vi "DriveModuleControl_TravTunePID.vi"(8 "error in":errorcluster, 9 "Actual State":T1={"Speed"=0.0, "Angle"={"VALUE"=0.0, "COS"=1.0, "SIN"=0.0}} {"Angle"."SIN" format="%13.4f"; "Angle"."COS" format="%13.4f"; "Angle"."VALUE" format="%13.4f"}, 10 "Desired State":T1={"Speed"=0.0, "Angle"={"VALUE"=0.0, "COS"=1.0, "SIN"=0.0}} {"Angle"."SIN" format="%13.4f"; "Angle"."COS" format="%13.4f"; "Angle"."VALUE" format="%13.4f"}, 11 "ModualNamePrefix":i32) -> (0 "error out":errorcluster)   [LabVIEW 2023]
uses:
  <vilib>/Rock Robotics/WPI/ThirdParty/JAS_Junk/TrajLib/TypeDef/SWERVE_DRIVE_MODULE_STATE.ctl
  <vilib>/Rock Robotics/WPI/ThirdParty/JAS_Junk/TrajLib/TypeDef/ROTATION2D.ctl
  <vilib>/Rock Robotics/WPI/ThirdParty/JAS_Junk/TrajLib/Rotation2d_Minus.vi
  <vilib>/Rock Robotics/WPI/ThirdParty/JAS_Junk/TrajLib/Rotation2d_GetRadians.vi
  <vilib>/Rock Robotics/WPI/ThirdParty/JAS_Junk/TrajLib/SwerveModuleState_New.vi
  <vilib>/Rock Robotics/WPI/ThirdParty/JAS_Junk/TrajLib/Rotation2d_RotateBy.vi
  <vilib>/Rock Robotics/WPI/ThirdParty/JAS_Junk/TrajLib/Rotation2d_CreateAngle.vi
  <vilib>/Rock Robotics/WPI/ThirdParty/JAS_Junk/TrajLib/SimpleMotorFF_Calculate.vi
  <vilib>/Rock Robotics/WPI/ThirdParty/JAS_Junk/TrajLib/PIDController_AtSetpoint.vi
  <vilib>/Rock Robotics/WPI/ThirdParty/JAS_Junk/TrajLib/PIDController_SetPIDF.vi
  <vilib>/Rock Robotics/WPI/ThirdParty/JAS_Junk/TrajLib/PIDController_SetDerivativeFilter.vi
  <vilib>/Rock Robotics/WPI/ThirdParty/JAS_Junk/TrajLib/PIDController_SetIntegratorRange.vi
  <vilib>/Rock Robotics/WPI/ThirdParty/JAS_Junk/TrajLib/PIDController_SetTolerancePandV.vi
  <vilib>/Rock Robotics/WPI/ThirdParty/JAS_Junk/TrajLib/PIDController_DisableContinousInput.vi
  <vilib>/Rock Robotics/WPI/ThirdParty/JAS_Junk/TrajLib/PIDController_EnableContinousInput.vi
  <vilib>/Rock Robotics/WPI/ThirdParty/JAS_Junk/TrajLib/PIDController_Reset.vi
  <vilib>/Rock Robotics/WPI/ThirdParty/JAS_Junk/TrajLib/PIDController_New.vi
  <vilib>/Rock Robotics/WPI/ThirdParty/JAS_Junk/TrajLib/PIDController_SetOutputLimits.vi
  <vilib>/Rock Robotics/WPI/ThirdParty/JAS_Junk/TrajLib/Rotation2d_UnaryMinus.vi
  <vilib>/Rock Robotics/WPI/ThirdParty/JAS_Junk/TrajLib/Rotation2d_CreateXY.vi
  <vilib>/Rock Robotics/WPI/ThirdParty/JAS_Junk/TrajLib/PIDController_NewPeriod.vi
  <vilib>/Rock Robotics/WPI/ThirdParty/JAS_Junk/TrajLib/Util_CalcDist.vi
  <vilib>/Rock Robotics/SystemInterfaces/NetworkCommunication/NetComm_UsageReport_report.vi
  DriveGlobal.vi
  <vilib>/Rock Robotics/WPI/ThirdParty/JAS_Junk/TrajLib/Globals/Util_LibraryGlobals.vi
  <vilib>/Rock Robotics/WPI/ThirdParty/JAS_Junk/TrajLib/PIDController_AdvCalculate_FF_Sp_Pv.vi
  <vilib>/Rock Robotics/Network Tables/NT Write Number.vi
  <vilib>/Rock Robotics/WPI/ThirdParty/JAS_Junk/TrajLib/Trajectory_Library.lvlib
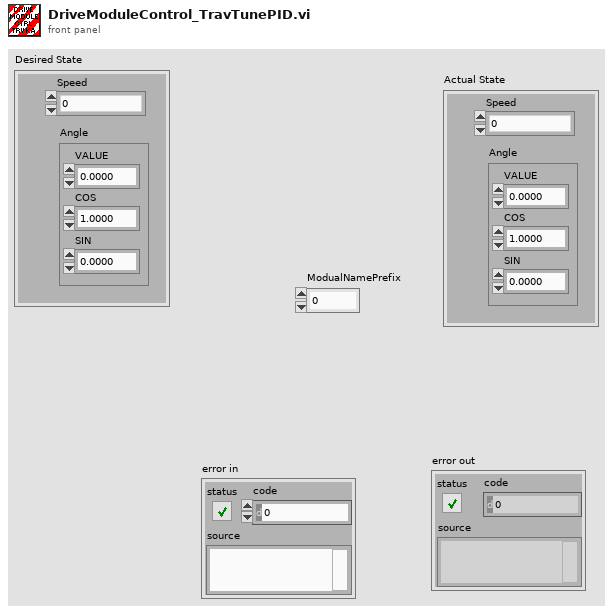
[diagram p1: front panel]
types:
  T1 = typedef "Trajectory_Library.lvlib/SWERVE_DRIVE_MODULE_STATE.ctl" = cluster{"Speed":dbl, "Angle":T2}
  T2 = typedef "Trajectory_Library.lvlib/ROTATION2D.ctl" = cluster{"VALUE":dbl, "COS":dbl, "SIN":dbl}
  T3 = enum16{"Ziegler Nicols - Fast", "Ziegler Nicols - Normal", "Ziegler Nicols - Slow", "CHR regulator - 0% overshoot", "CHR regulator - 20% overshoot", "CHR servo - 0 % overshoot", "CHR servo - 20% overshoot"}
  T4 = typedef "WPI_MotorControlDeviceRef.ctl" = cluster{"DeviceStatus":errorcluster, "Type":T5, "PWM":cluster{"PWM Channel":T6, "DeadBand":T7}, "CAN":cluster{"Device Number":u8, "SetOutput VI Ref":variant, "GetOutput VI Ref":variant, "Enable VI Ref":variant, "Disable VI Ref":variant, "Data":variant}, "Invert":bool, "DIO PWM":cluster{"PWM \"Enable\" Channel":T6, "DIOChannel":T8, "PWM Rate":dbl}}
  T5 = typedef "WPI_MotorControlType.ctl" = enum16{"PWM", "CAN", "DIO PWM"}
  T6 = typedef "FPGA_DIOPWMChannel.ctl" = enum8{"PWM 0", "PWM 1", "PWM 2", "PWM 3", "PWM 4", "PWM 5", "PWM 6", "PWM 7", "PWM 8", "PWM 9", "PWM MXP 0", "PWM MXP 1", "PWM MXP 2", "PWM MXP 3", "PWM MXP 4", "PWM MXP 5", "PWM MXP 6", "PWM MXP 7", "PWM MXP 8", "PWM MXP 9", "Invalid"}
  T7 = typedef "WPI_PWMDeadband.ctl" = cluster{"Name":string, "maxPositivePwm":i32, "minPositivePwm":i32, "centerPwm":i32, "maxNegativePwm":i32, "minNegativePwm":i32, "angularRange":u16}
  T8 = typedef "FPGA_DIOChannel.ctl" = enum8{"DIO 0", "DIO 1", "DIO 2", "DIO 3", "DIO 4", "DIO 5", "DIO 6", "DIO 7", "DIO 8", "DIO 9", "DIO MXP 0", "DIO MXP 1", "DIO MXP 2", "DIO MXP 3", "DIO MXP 4", "DIO MXP 5", "DIO MXP 6", "DIO MXP 7", "DIO MXP 8", "DIO MXP 9", "DIO MXP 10", "DIO MXP 11", "DIO MXP 12", "DIO MXP 13", "DIO MXP 14", "DIO MXP 15", "SPI Port CS1", "SPI Port CS2", "SPI Port CS3", "SPI Port MISO", "SPI Port MOSI", "Invalid"}
  T9 = typedef "Trajectory_Library.lvlib/SIMPLE_MOTOR_FF.ctl" = cluster{"Ks":dbl, "Kv":dbl, "Ka":dbl, "KnInv":dbl}
  T10 = typedef "Trajectory_Library.lvlib/PID_ADV_LIMITS.ctl" = cluster{"MaxInput":dbl, "MinInput":dbl, "Continuous":bool, "MaxOutput":dbl, "MinOutput":dbl}
  T11 = typedef "Trajectory_Library.lvlib/PID_ADV_TUNING.ctl" = cluster{"Kf":dbl, "Kp":dbl, "Ki":dbl, "Kd":dbl, "MaximumIntegral":dbl, "MinimumIntegral":dbl, "Filter Derivative":bool}
  T12 = cluster{"Controller Constant Type":enum16{"Ziegler Nicols - Fast", "Ziegler Nicols - Normal", "Ziegler Nicols - Slow", "CHR regulator - 0% overshoot", "CHR regulator - 20% overshoot", "CHR servo - 0 % overshoot", "CHR servo - 20% overshoot"}, "Type of Controller":enum16{"P", "PI", "PID"}, "CO Offset":dbl, "Kn":dbl, "Tuning Tolerance":dbl, "Plant Tolerance":dbl, "Newest Avg Time ":i32, "Long Ave Time":i32}
  T13 = cluster{"Plant Gain (K)":dbl, "Time Constant (T)":dbl, "Dead Time (L)":dbl, "stimulus operating point":dbl, "response operating point":dbl}
  T14 = cluster{"proportional gain (Kp)":dbl, "integral time (Ki / Sec)":dbl, "derivative time (Kd /Sec)":dbl}
  T15 = cluster{"Const Done":bool, "Plant Done":bool, "PV Std Dev":dbl, "CO Std Dev":dbl}
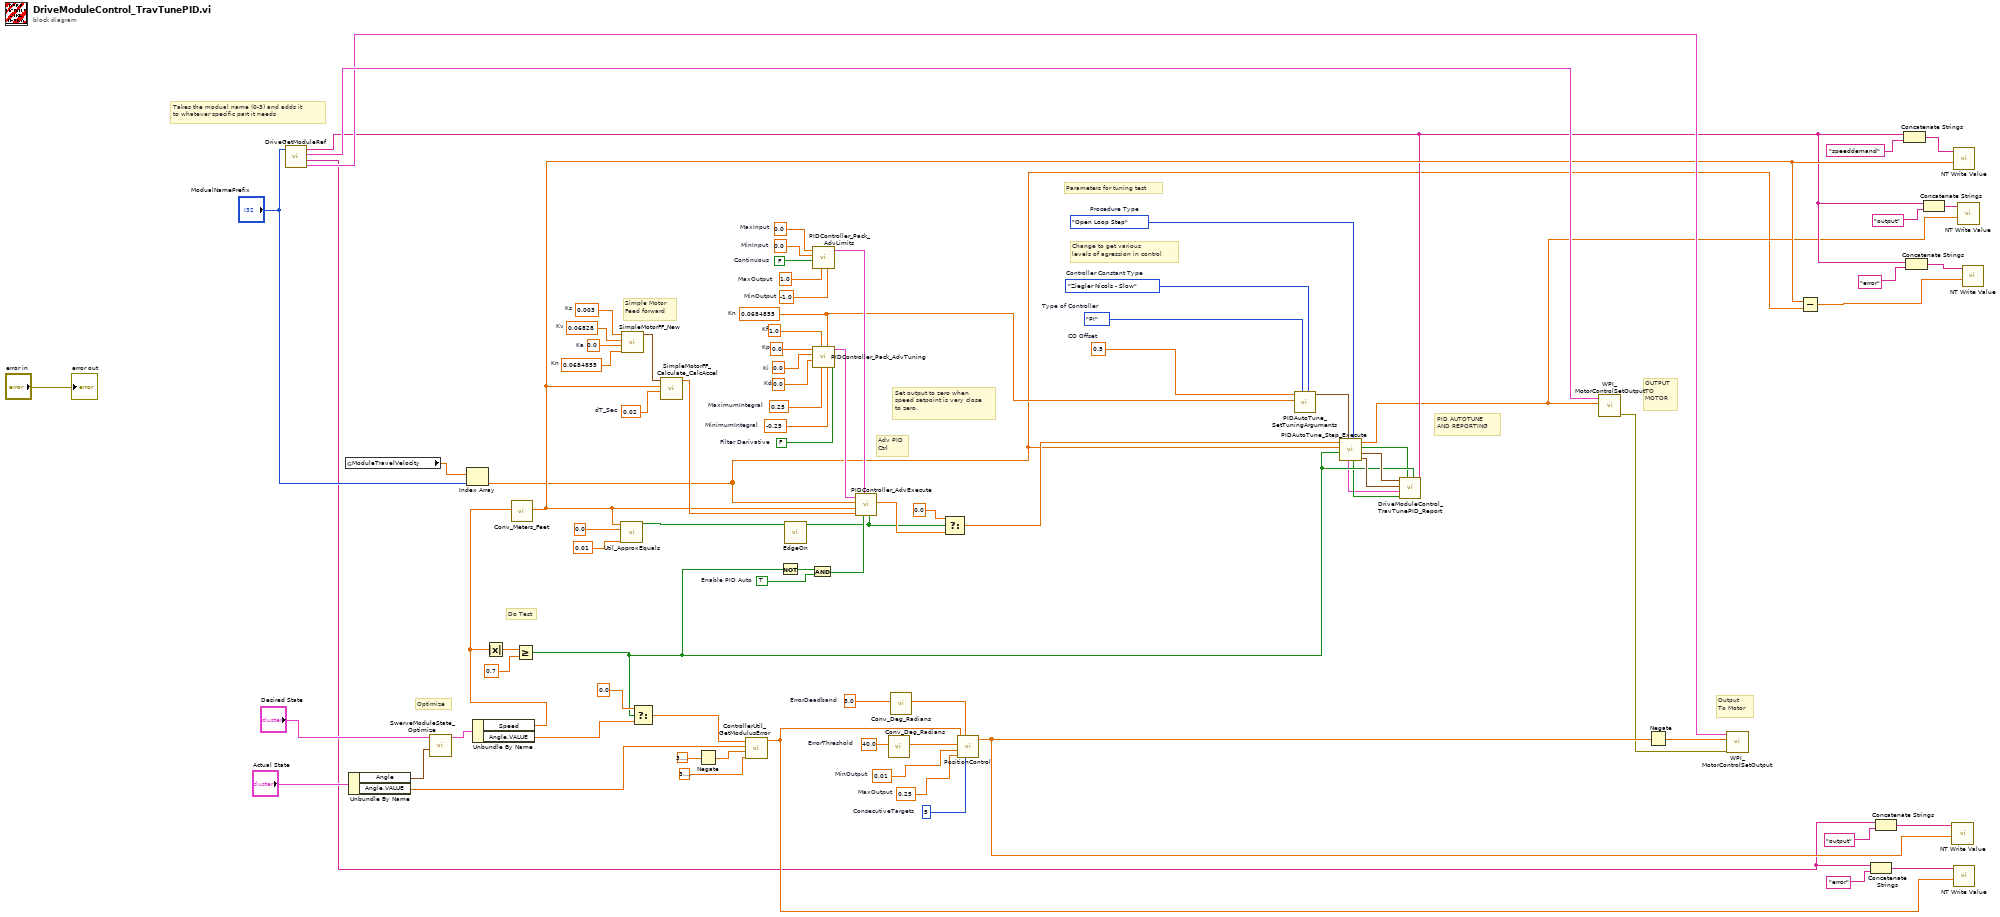
[diagram p0: block diagram]
diagram:
  w12 = enum16{"Open Loop Step", "Closed Loop Step"}."Open Loop Step"  # Procedure Type
  w13 = T3."Ziegler Nicols - Slow"  # Controller Constant Type
  w14 = enum16{"P", "PI", "PID"}."PI"  # Type of Controller
  w15 = 0.5  # CO Offset
  w27 = TRUE  # Enable PID Auto
  w11 = 0.0684855  # Kn
  w53 = 0.0  # Kp
  w52 = 0.0  # Ki
  w51 = 0.0  # Kd
  w50 = 1.0  # Kf
  w49 = 0.25  # MaximumIntegral
  w48 = -0.25  # MinimumIntegral
  w47 = FALSE  # Filter Derivative
  w45 = 0.0  # MinInput
  w44 = FALSE  # Continuous
  w43 = 1.0  # MaxOutput
  w46 = -1.0  # MinOutput
  w42 = 0.0  # MaxInput
  w62 = 0.0684855  # Kn
  w61 = 0.02  # dT_Sec
  w59 = 0.003  # Ks
  w58 = 0.06828  # Kv
  w57 = 0.0  # Ka
  w72 = 5  # ConsecutiveTargets
  w69 = 0.25  # MaxOutput
  w73 = 0.01  # MinOutput
  w66 = 40.0  # ErrorThreshold
  w68 = 3.0  # ErrorDeadband
  # "Output\nTo Motor"
  # "OUTPUT\nTO \nMOTOR"
  # "PID AUTOTUNE\nAND REPORTING"
  # "Change to get various\nlevels of agression in control"
  # "Parameters for tuning test"
  # "Do Test"
  # "Optimize"
  # "Set output to zero when\nspeed setpoint is very close\nto zero."
  # "Adv PID\nCtrl"
  # "Simple Motor\nFeed forward"
  # "Takes the modual name (0-3) and adds it \nto whatever specific part it needs"
  n1 = call "DriveGetModuleRef.vi"("ModualNamePrefix"="ModualNamePrefix") -> ("SpinMot"=w54:T4, "SpinStr"=w33:string, "TravMot"=w55:T4, "TravStr"=w5:string)  [unwired: 5 in, 2 out]
  n2 = global read "DriveGlobal.vi" "ModuleTravelVelocity"() -> (w38:dbl[])
  n3 = Unbundle By Name("Actual State") -> ("Angle"=w79:T2, "Angle.VALUE"=w76:dbl)
  n4 = call <vilib>:"SwerveModuleState_Optimize.vi"("CurrentAngle"=w79, "Desired State"="Desired State") -> ("out SWERVE_DRIVE_MODULE_STATE"=w77:T1)  [unwired: 9 in]
  n5 = Index Array(array=w38, index="ModualNamePrefix") -> (element=w1:dbl)
  n6 = Unbundle By Name(w77) -> ("Speed"=w24:dbl, "Angle.VALUE"=w21:dbl)
  n7 = Absolute Value(x=w24) -> (abs(x)=w23:dbl)
  n8 = call <vilib>:"Conv_Meters_Feet.vi"("Meters"=w24) -> ("Feet"=w30:dbl)  [unwired: 10 in]
  n9 = Greater Or Equal?(x=w23, y=0.7) -> (x >= y?=w7:bool)
  n10 = call <vilib>:"Util_ApproxEquals.vi"("Tolerance"=0.01, "Value 2"=0.0, "Value 1"=w30) -> ("ApproxEquals"=w18:bool)  [unwired: 8 in]
  n11 = call <vilib>:"SimpleMotorFF_New.vi"("Kn"=w62, "Ka"=w57, "Kv"=w58, "Ks"=w59) -> ("SIMPLE_MOTOR_FF"=w60:T9)  [unwired: 7 in]
  n12 = Select(t=0.0, s=w7, f=w21) -> (s? t:f=w19:dbl)
  n13 = call <vilib>:"SimpleMotorFF_Calculate_CalcAccel.vi"("dT_Sec"=w61, "VelSp"=w30, "SIMPLE_MOTOR_FF"=w60) -> ("FeedForward"=w39:dbl)  [unwired: 8 in]
  n14 = Negate(x=3.141592653589793) -> (-x=w78:dbl)
  n15 = call <vilib>:"ControllerUtil_GetModulusError.vi"("Maximum_Input"=3.141592653589793, "Minimum_Input"=w78, "Measurerment(PV)"=w76, "Reference(SP)"=w19) -> ("Error"=w70:dbl)  [unwired: 7 in]
  n16 = Not(x=w7) -> (.not. x?=w28:bool)
  n17 = call "EdgeOn.vi"("Current State"=w18) -> ("Edge On Found"=w17:bool)  [unwired: 10 in]
  n18 = And(x=w28, y=w27) -> (x .and. y?=w29:bool)
  n19 = call <vilib>:"PIDController_Pack_AdvLimits.vi"("MinOutput"=w46, "MaxOutput"=w43, "Continuous"=w44, "MinInput"=w45, "MaxInput"=w42) -> ("Adv PID Limits"=w40:T10)  [unwired: 6 in]
  n20 = call <vilib>:"PIDController_Pack_AdvTuning.vi"("Filter Derivative"=w47, "MinimumIntegral"=w48, "Kn"=w11, "MaximumIntegral"=w49, "Kf"=w50, "Kd"=w51, "Ki"=w52, "Kp"=w53) -> ("Adv PID Tuning"=w41:T11)  [unwired: 3 in]
  n21 = call <vilib>:"PIDController_AdvExecute.vi"("Reset"=w17, "Auto"=w29, "Adv PID Limits"=w40, "FF-FeedForward"=w39, "SP-SetPoint"=w30, "PV-Measurement"=w1, "Adv PID Tuning"=w41) -> ("CO-ControlOutput"=w26:dbl)  [unwired: 2 in, 2 out]
  n22 = call <vilib>:"Conv_Deg_Radians.vi"("Degress"=w66) -> ("Radians"=w65:dbl)  [unwired: 10 in]
  n23 = call <vilib>:"Conv_Deg_Radians.vi"("Degress"=w68) -> ("Radians"=w67:dbl)  [unwired: 10 in]
  n24 = Select(t=0.0, s=w17, f=w26) -> (s? t:f=w10:dbl)
  n25 = call "PositionControl.vi"("ConsecutiveTargets"=w72, "ErrorDeadband"=w67, "MaxOutput"=w69, "MinOutput"=w73, "ErrorThreshold"=w65, "Error"=w70) -> ("OutputValue"=w64:dbl)  [unwired: 3 in, 2 out]
  n26 = call <vilib>:"PIDAutoTune_SetTuningArguments.vi"("Controller Constant Type"=w13, "Type of Controller"=w14, "Kn"=w11, "CO Offset"=w15) -> ("Configuration Parameters"=w16:T12)  [unwired: 7 in]
  n27 = call <vilib>:"PIDAutoTune_Step_Execute.vi"("Procedure Type"=w12, "Configuration Parameters"=w16, "Tune"=w7, "Measurement  (PV)"=w1, "Control Output (Co)"=w10) -> ("Plant and Test Data"=w8:T13, "New Tuning Parameters"=w9:T14, "Tuning Done"=w6:bool, "Adj CO"=w2:dbl, "Error Occured"=w4:bool, "Diagnostic Info"=w3:T15)  [unwired: 1 in]
  n28 = call "DriveModuleControl_TravTunePID_Report.vi"("Network Table Prefix"=w5, "TestInProgress"=w7, "Tuning Done"=w6, "Error Occured"=w4, "Diagnostic Info"=w3, "Plant and Test Data"=w8, "New Tuning Parameters"=w9) -> ()  [unwired: 5 in]
  n29 = call <vilib>:"WPI_MotorControlSetOutput.vi"("Output"=w2, "MotorControlDevRef"=w55) -> ("error out"=w56:errorcluster)  [unwired: 7 in, 2 out]
  n30 = Negate(x=w64) -> (-x=w63:dbl)
  n31 = call <vilib>:"WPI_MotorControlSetOutput.vi"("error in (no error)"=w56, "Output"=w63, "MotorControlDevRef"=w54) -> ()  [unwired: 6 in, 3 out]
  n32 = Subtract(x=w30, y=w1) -> (x-y=w34:dbl)
  n33 = Concatenate Strings(w33, "error" ("refnum name")) -> (w83:string)
  n34 = Concatenate Strings(w33, "output" ("refnum name")) -> (w71:string)
  n35 = Concatenate Strings(w5, "speeddemand" ("refnum name")) -> (w87:string)
  n36 = Concatenate Strings(w5, "error" ("refnum name")) -> (w35:string)
  n37 = Concatenate Strings(w5, "output" ("refnum name")) -> (w85:string)
  n38 = call-poly <vilib>:"NT Write Value.vi"("value"=w64, "name"=w71) -> ()  [unwired: 9 in, 1 out]
  n39 = call-poly <vilib>:"NT Write Value.vi"("value"=w30, "name"=w87) -> ()  [unwired: 9 in, 1 out]
  n40 = call-poly <vilib>:"NT Write Value.vi"("value"=w70, "name"=w83) -> ()  [unwired: 9 in, 1 out]
  n41 = call-poly <vilib>:"NT Write Value.vi"("value"=w2, "name"=w85) -> ()  [unwired: 9 in, 1 out]
  n42 = call-poly <vilib>:"NT Write Value.vi"("value"=w34, "name"=w35) -> ()  [unwired: 9 in, 1 out]
  "error out" <- "error in"
